vi "blob.vi"   [LabVIEW 2012]
uses:
  <vilib>/addons/internet/NI_InternetTK_Core_VIs.lvlib
  <vilib>/addons/internet/NI_InternetTK_Common_VIs.lvlib
types:
  T1 = typedef "CGI Connection Info.ctl" = cluster{"name":string, "type":T2, "session":T3}
  T2 = typedef "CGI Request Type.ctl" = enum16{"cgi", ".spool first", ".spool", ".spool last"}
  T3 = typedef "HTTP Session.ctl" = refnum<k1>
  T4 = typedef "Cookie.ctl" = cluster{"cookie id":string, "address":string}
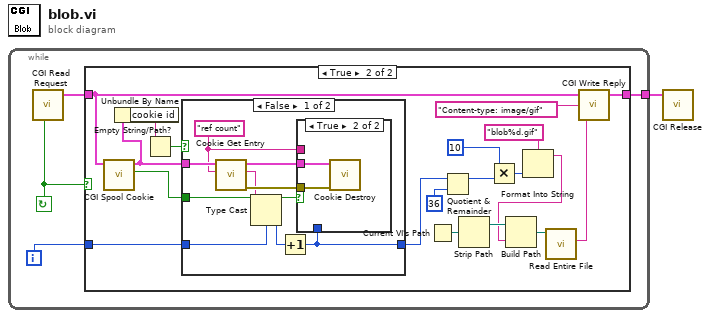
[diagram p0: block diagram]
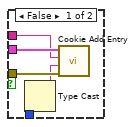
[diagram p3: hidden frame]
diagram:
  n1 = while {
    tunnel: [w5] -> w1
    i -> [w4]
    stop <- w2 continue-if-true
    n2 = call <vilib>:"CGI Read Request.vi"() -> ("valid request?"=w2:bool, "cgi connection info"=w3:T1)  [unwired: 4 in, 2 out]
    n3 = case shown="True" w2 {
      tunnel: [w6 w25] -> w5
      tunnel: w3 -> [w6 w8]
      tunnel: w4 -> [_ w15]
      frame False {
      }
      frame True {
        n4 = call <vilib>:"CGI Spool Cookie.vi"("cgi connection info"=w8) -> ("destroy cookie?"=w7:bool, "cookie"=w10:T4)  [unwired: 7 in, 2 out]
        n5 = Unbundle By Name(w10) -> ("cookie id"=w9:string)
        n6 = Empty String/Path?(string/path=w9) -> (empty?=w13:bool)
        n7 = case shown="False" w13 {
          tunnel: w15 -> [w29 w42]
          tunnel: [w32 w42] -> w12
          tunnel: w10 -> [w34 _]
          tunnel: w7 -> [w27 _]
          frame False {
            w31 = "ref count" ("key")
            n8 = call <vilib>:"Cookie Get Entry.vi"("key"=w31, "cookie"=w34) -> ("error out"=w28:errorcluster, "value"=w26:string, "cookie out"=w30:T4)  [unwired: 2 in, 1 out]
            n9 = Type Cast(type=w29, x=w26) -> (*(type *) &x=w33:i32)
            n10 = Increment(x=w33) -> (x+1=w32:i32)
            n11 = case shown="True" w27 {
              tunnel: w28 -> [w39 w41]
              tunnel: w30 -> [w36 w40]
              tunnel: w31 -> [w35 _]
              tunnel: w32 -> [w38 _]
              frame False {
                n12 = Type Cast(x=w38) -> (*(type *) &x=w37:string)  [unwired: 1 in]
                n13 = call <vilib>:"Cookie Add Entry.vi"("error in (no error)"=w39, "value"=w37, "key"=w35, "cookie"=w36) -> ()  [unwired: 4 out]
              }
              frame True {
                n14 = call <vilib>:"Cookie Destroy.vi"("error in (no error)"=w41, "cookie"=w40) -> ()  [unwired: 8 in, 2 out]
              }
            }
          }
          frame True {
          }
        }
        n15 = Current VI's Path() -> (path=w21:path)
        n16 = Quotient & Remainder(x=w12, y=36) -> (x-y*floor(x/y)=w14:i32)  [unwired: 1 out]
        n17 = Strip Path(path=w21) -> (stripped path=w20:path)  [unwired: 1 out]
        n18 = Multiply(x=10, y=w14) -> (x*y=w22:i32)
        n19 = Format Into String(format string="blob%d.gif", w22) -> (resulting string=w19:string)  [unwired: 2 in, 1 out]
        n20 = Build Path(base path=w20, name or relative path=w19) -> (appended path=w18:path)
        n21 = call <vilib>:"Read Entire File.vi"("path"=w18) -> ("data"=w17:string)  [unwired: 7 in, 3 out]
        n22 = call <vilib>:"CGI Write Reply.vi"("content"=w17, "header"="Content-type: image/gif", "cgi connection info"=w8) -> ("cgi connection info out"=w25:T1)  [unwired: 2 in]
      }
    }
  }
  n23 = call <vilib>:"CGI Release.vi"("cgi connection info"=w1) -> ()  [unwired: 5 in]
